vi "Run ESC Flight Profile.vi"(9 "Flight Profile File":path, 10 "Simulate/Run":T1=enum."Run VI", 11 "RPM PWM Calib File":path) -> (0 "error IO":errorcluster, 1 "Flight Profile Out":path)   [LabVIEW 2021]
uses:
  Anemometry/Anemometry Sub Vis/Controls/User_Specific_mode.ctl
  Anemometry/Anemometry Sub Vis/Controls/Inst_type.ctl
  Anemometry/Anemometry Sub Vis/Gen Trav/Multi_Run_Status.ctl
  Anemometry/Anemometry Sub Vis/Globals/Trav_pos_global.vi
  Anemometry/Anemometry Sub Vis/Globals/Meas_global.vi
panel:
  out "PWM":dbl format="%.2f"
  out "Time (s)":dbl[](array[numeric])
  out "Calib Constants":dbl[](array[numeric])
  out "XY Graph":cluster{dbl[], dbl[]}(graph)
  out "RPM":dbl[](array[numeric])
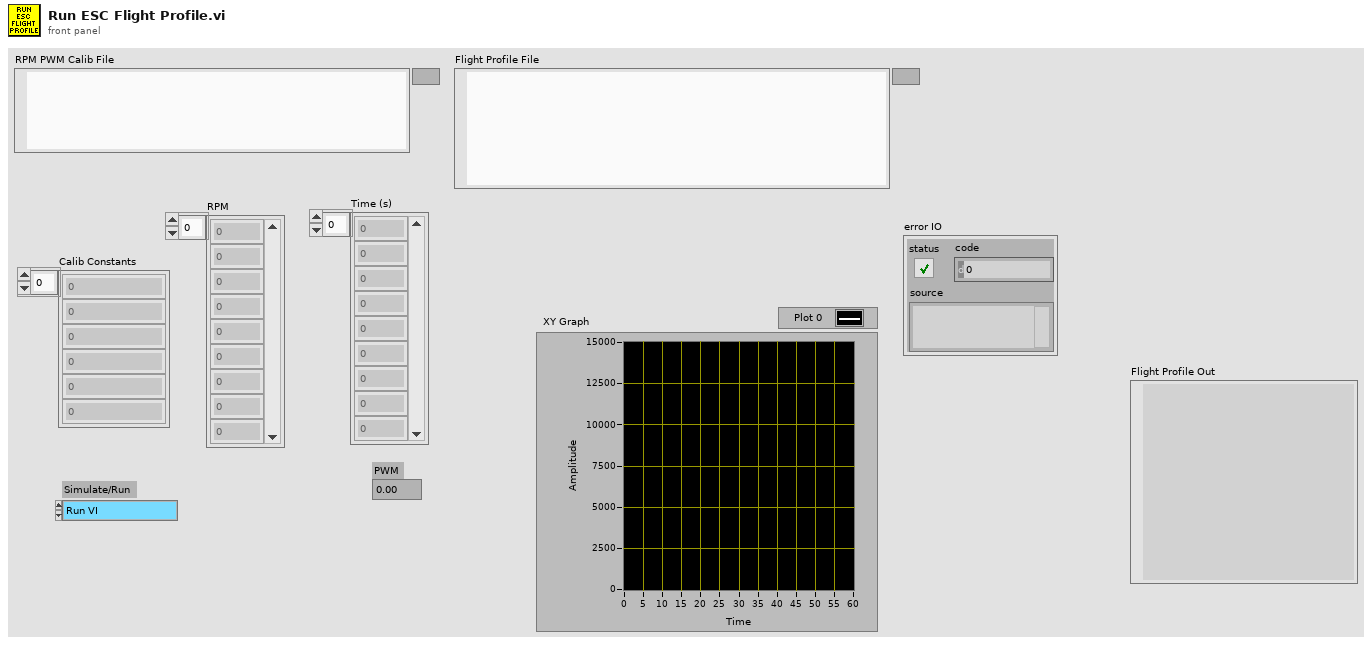
[diagram p1: front panel]
types:
  T1 = typedef "User_Specific_mode.ctl" = enum16{"Check VI only", "Run VI"}
  T2 = typedef "Inst_type.ctl" = enum16{"Raw voltage", "Raw with zero offsetting", "Propeller anemometer", "Pressure Transducer", "Pitot-static tube", "Hot wire", "Cross wire 1", "Cross wire 2", "Generic Linear", "Generic Polynomial", "Generic BackPoly", "Fast FID", "Thermocouple", "Cold wire", "Pulsed Wire", "LDA Vel", "LDA Tran time", "LDA Arr time", "Microphone"}
  T3 = typedef "Multi_Run_Status.ctl" = enum16{"Continue", "Continue with Error", "Jump to Next Point", "Jump to Next Row", "Jump To Fall Back", "Terminate Run"}
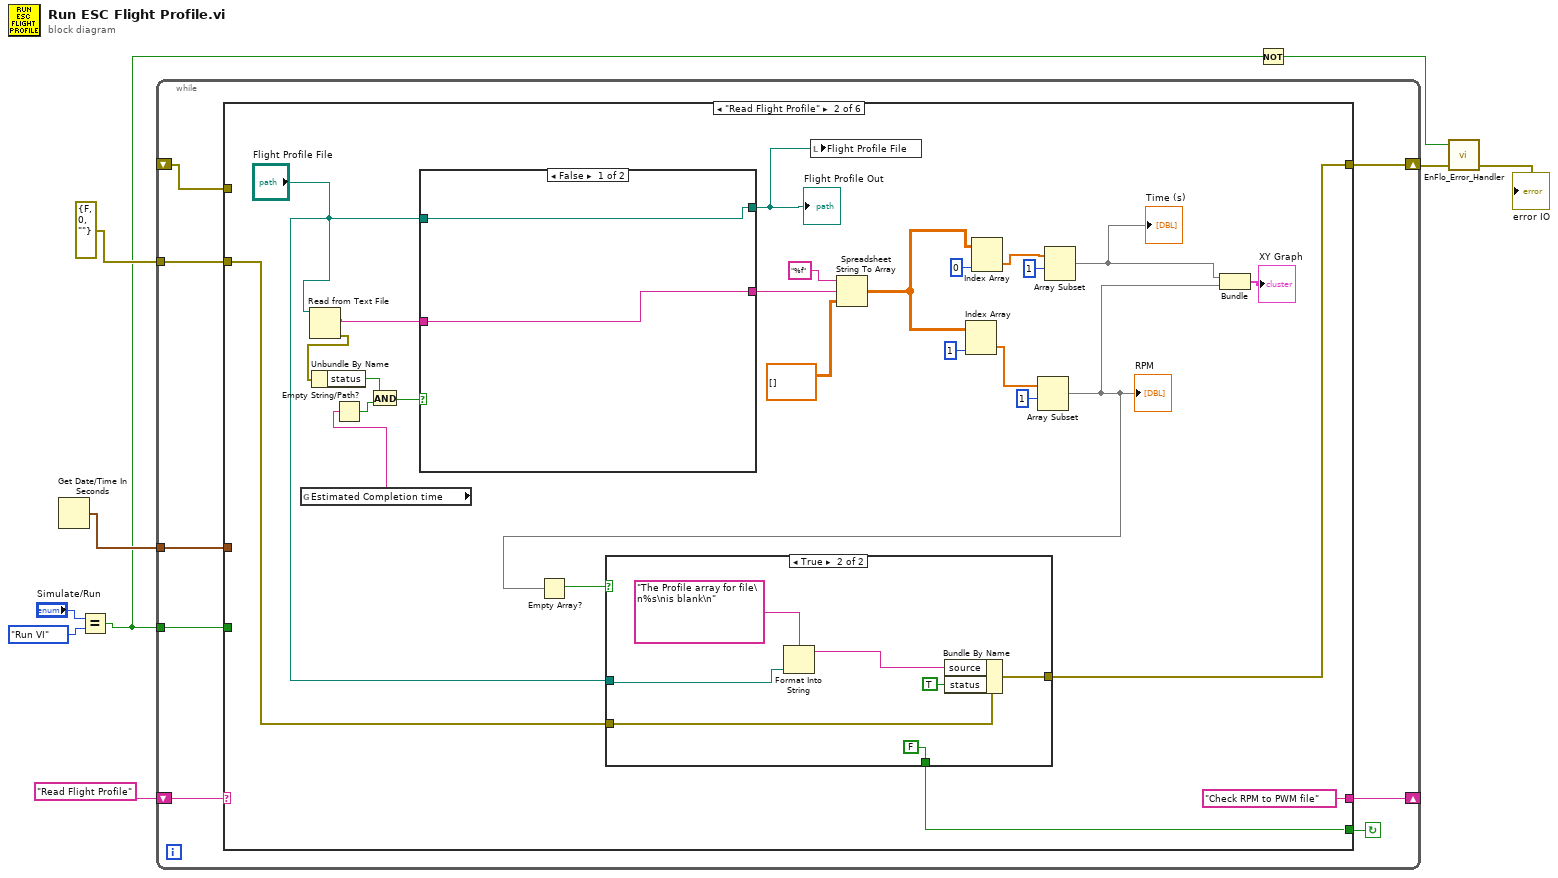
[diagram p0: block diagram]
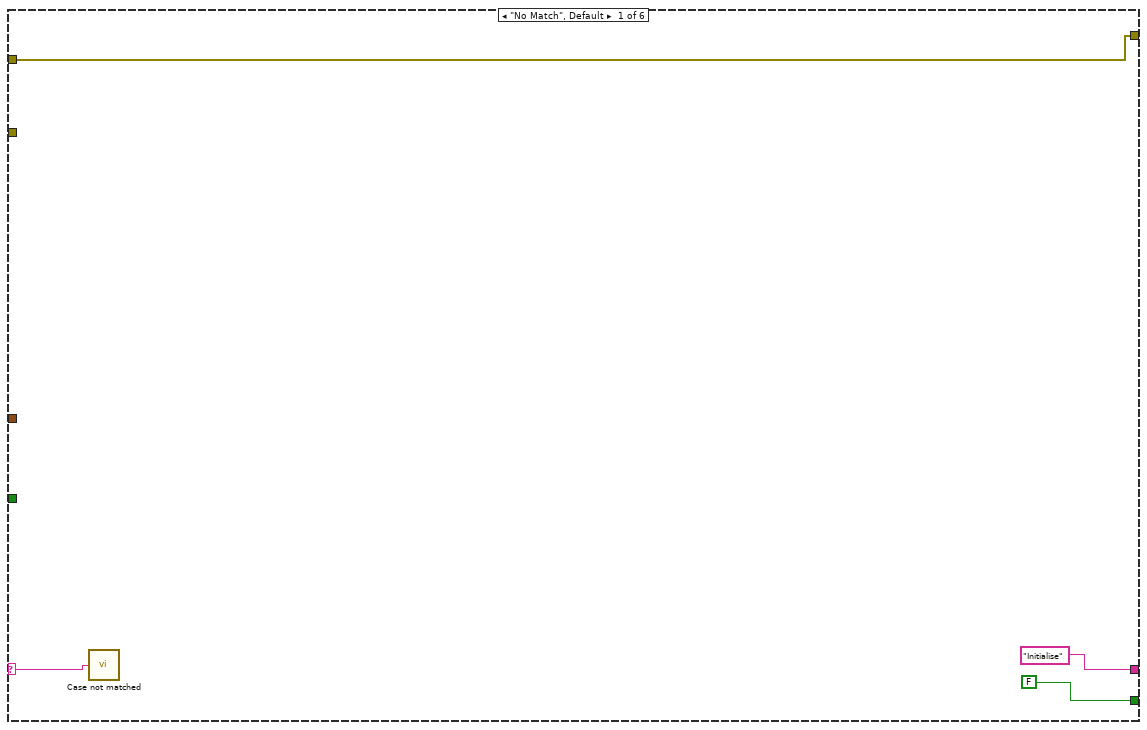
[diagram p2: hidden frame]
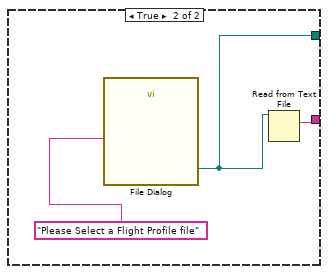
[diagram p3: hidden frame]
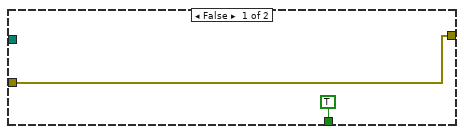
[diagram p4: hidden frame]
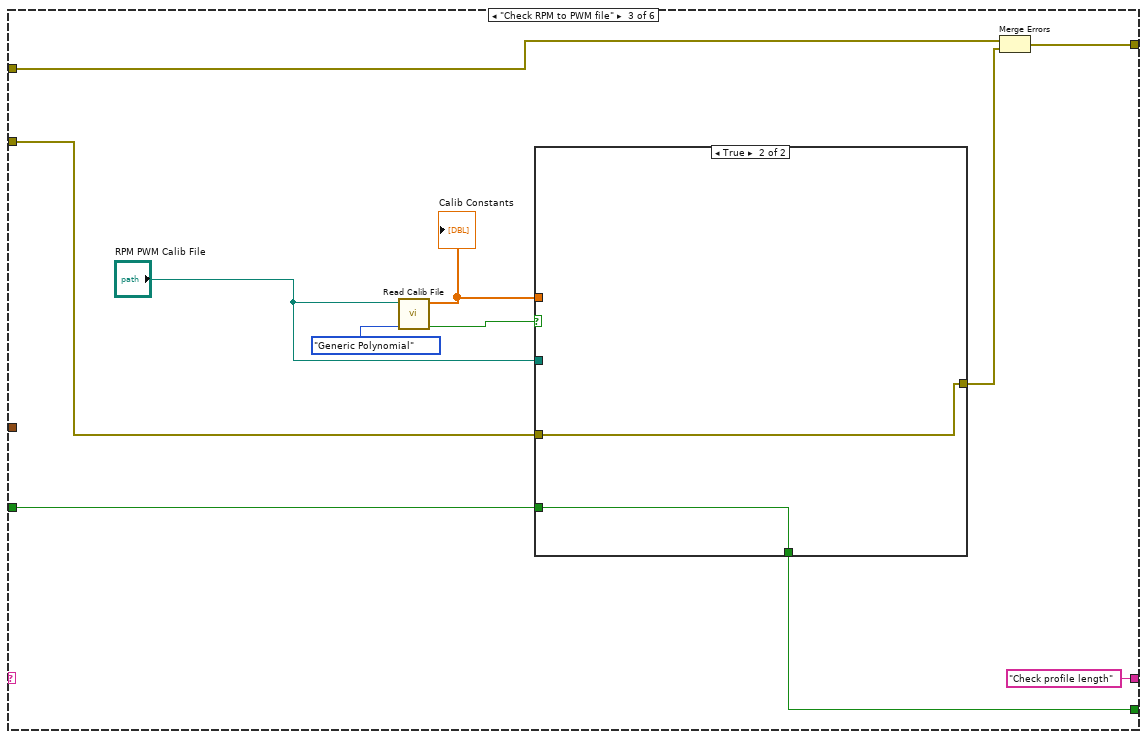
[diagram p5: hidden frame]
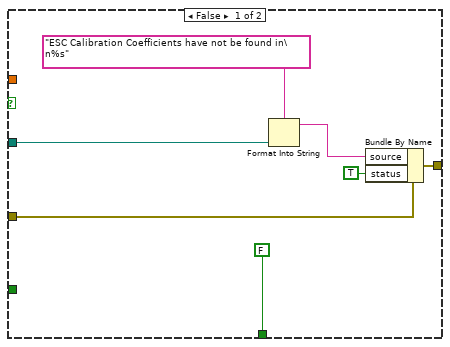
[diagram p6: hidden frame]
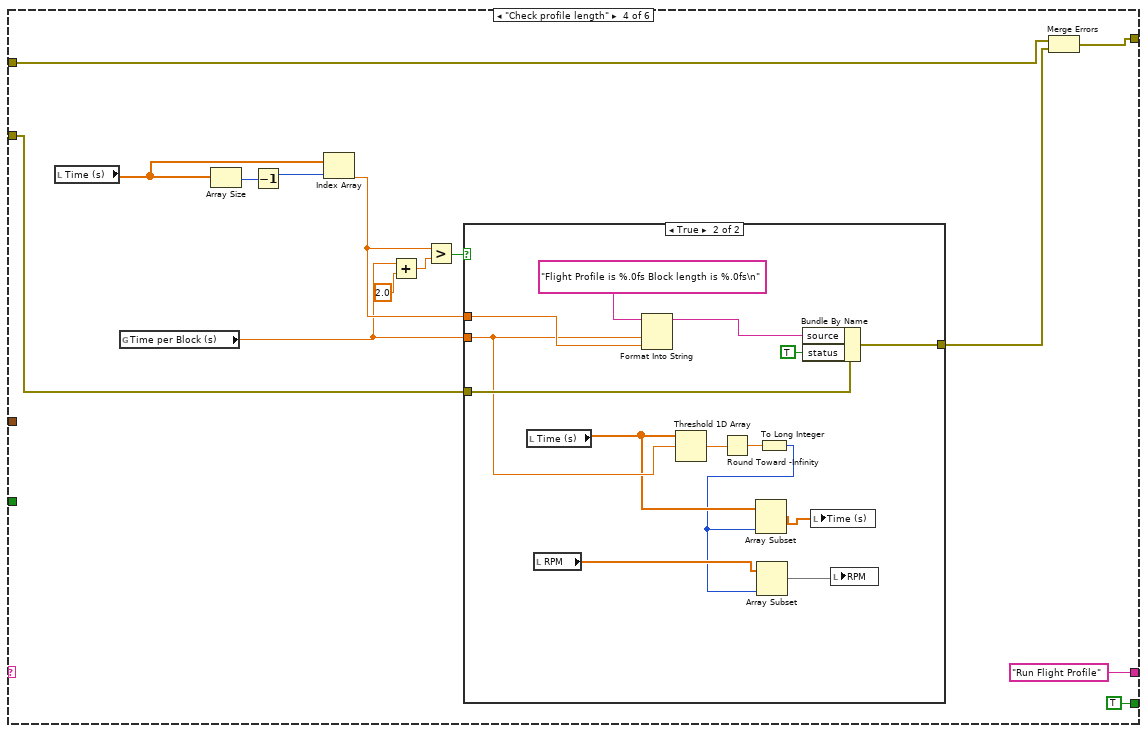
[diagram p7: hidden frame]
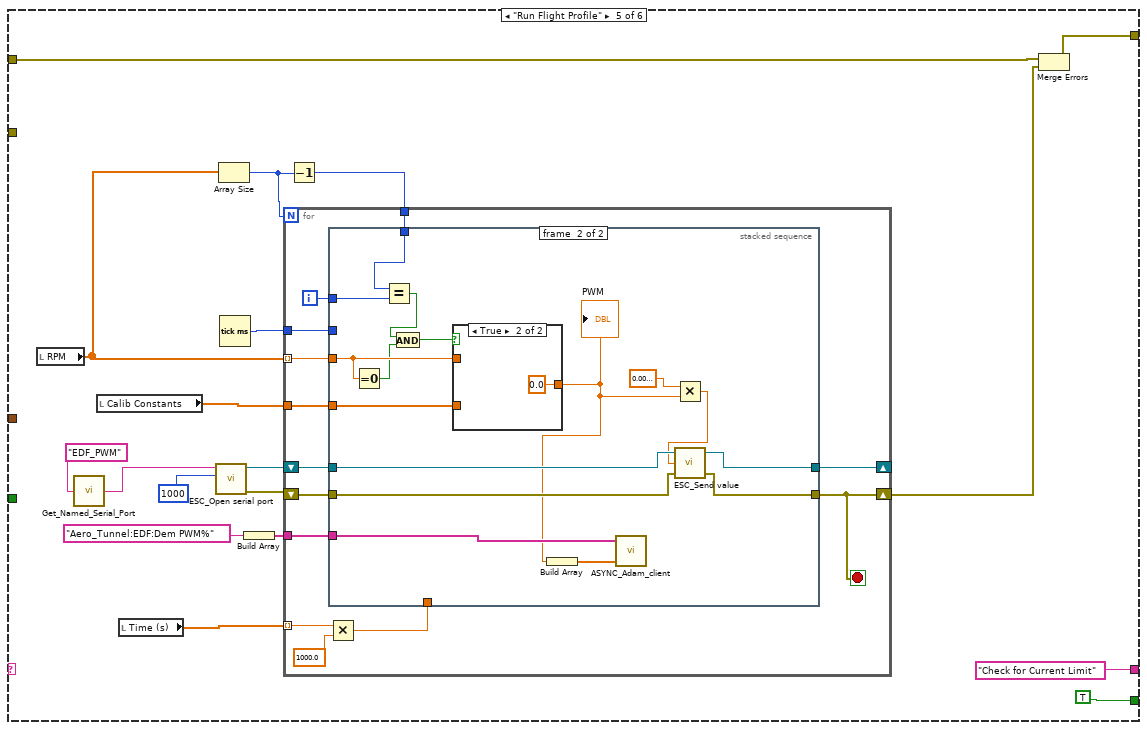
[diagram p9: hidden frame]
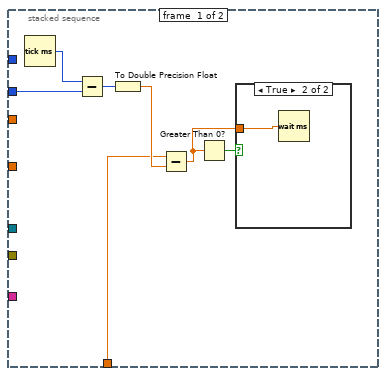
[diagram p10: hidden frame]
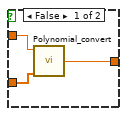
[diagram p12: hidden frame]
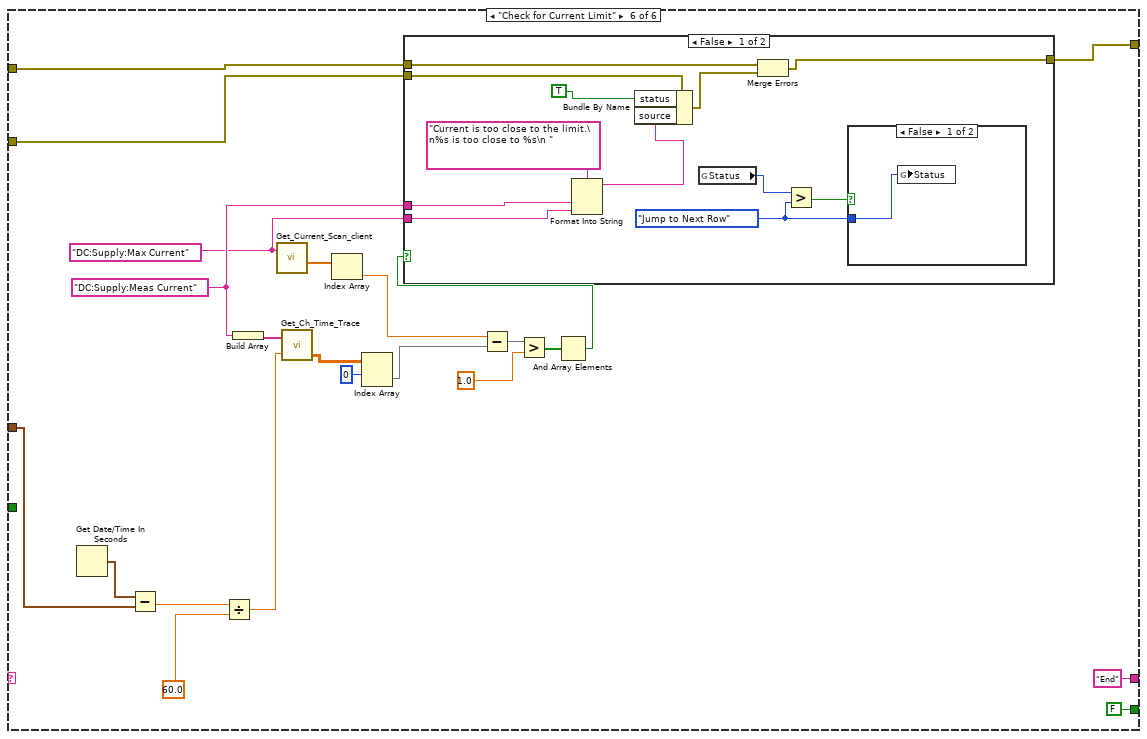
[diagram p13: hidden frame]
diagram:
  n1 = Get Date/Time In Seconds() -> (seconds since 1Jan1904=w7:timestamp)
  n2 = Equal?(x="Simulate/Run", y=User_Specific_mode."Run VI" ("Simulate/Run")) -> (x = y?=w2:bool)
  n3 = while {
    shift-left: "Read Flight Profile" -> [w14]
    shift-right: [w15] -> _
    tunnel: w7 -> [w13]
    tunnel: errorcluster {"status"=FALSE, "code"=0, "source"=""} ("error in (no error)") -> [w12]
    shift-right: [w11] -> w5
    shift-left: _ -> [w10]
    tunnel: w2 -> [w9]
    stop <- w16 continue-if-true
    n4 = case shown="\"Read Flight Profile\"" w14 {
      selector: w14 -> [w18 _ _ _ _ _]
      tunnel: [FALSE w34 w66 TRUE TRUE FALSE] -> w16
      tunnel: ["Initialise" "Check RPM to PWM file" "Check profile length" "Run Flight Profile" "Check for Current Limit" "End"] -> w15
      tunnel: w13 -> [_ _ _ _ _ w186]
      tunnel: w12 -> [_ w31 w64 w87 _ w171]
      tunnel: [w17 w30 w63 w84 w110 w169] -> w11
      tunnel: w10 -> [w17 _ w62 w85 w111 w170]
      tunnel: w9 -> [_ _ w61 _ _ _]
      frame "No Match", Default {
        n5 = call "Case not matched.vi"("Case Name not Matched"=w18) -> ()
      }
      frame "Read Flight Profile" {
        n6 = global read "Trav_pos_global.vi" "Estimated Completion time"() -> (w26:string)
        n7 = Read from Text File(file (use dialog)="Flight Profile File") -> (text=w23:string, error out=w29:errorcluster)  [unwired: 3 in, 2 out]
        n8 = Unbundle By Name(w29) -> ("status"=w28:bool)
        n9 = Empty String/Path?(string/path=w26) -> (empty?=w27:bool)
        n10 = And(x=w28, y=w27) -> (x .and. y?=w25:bool)
        n11 = case shown="False" w25 {
          tunnel: [w48 w50] -> w24
          tunnel: w23 -> [w48 _]
          tunnel: [w47 w49] -> w21
          tunnel: "Flight Profile File" -> [w47 _]
          frame False {
          }
          frame True {
            n12 = call "File Dialog"("prompt"="Please Select a Flight Profile file") -> ("selected path"=w49:path)  [unwired: 11 in, 3 out]
            n13 = Read from Text File(file (use dialog)=w49) -> (text=w50:string)  [unwired: 3 in, 3 out]
          }
        }
        "Flight Profile Out" <- w21
        n14 = local write "Flight Profile File"(w21) -> ()
        n15 = Spreadsheet String To Array(format string="%f", spreadsheet string=w24, array type (2D Dbl)=dbl[][] []) -> (array=w45:dbl[][])  [unwired: 1 in]
        n16 = Index Array(array=w45, index (col)=1 ("disabled index (col)")) -> (element=w44:dbl[])  [unwired: 1 in]
        n17 = Index Array(array=w45, index (col)=0 ("disabled index (col)")) -> (element=w46:dbl[])  [unwired: 1 in]
        n18 = Array Subset(array=w44, index=1) -> (w36:dbl[])  [unwired: 1 in]
        "RPM" <- w36
        n19 = Empty Array?(array=w36) -> (empty?=w35:bool)
        n20 = case shown="True" w35 {
          tunnel: [TRUE FALSE] -> w34
          tunnel: "Flight Profile File" -> [_ w59]
          tunnel: w31 -> [w52 w57]
          tunnel: [w52 w54] -> w30
          frame False {
          }
          frame True {
            n21 = Format Into String(format string="The Profile array for file\n%s\nis blank\n", w59) -> (resulting string=w55:string)  [unwired: 2 in, 1 out]
            n22 = Bundle By Name(cluster=w57, "source"=w55, "status"=TRUE) -> (w54:errorcluster)
          }
        }
        n23 = Array Subset(array=w46, index=1) -> (w32:dbl[])  [unwired: 1 in]
        "Time (s)" <- w32
        n24 = Bundle(w32, w36) -> (→"XY Graph":cluster{dbl[], dbl[]})  [unwired: 1 in]
      }
      frame "Check RPM to PWM file" {
        n25 = call "Read Calib File.vi"("Inst type"=Inst_type."Generic Polynomial", "Calib File"="RPM PWM Calib File") -> ("Coefficients Found?"=w68:bool, "Calib Constants"=w69:dbl[])  [unwired: 8 in]
        "Calib Constants" <- w69
        n26 = case shown="True" w68 {
          tunnel: w69 -> [_ _]
          tunnel: "RPM PWM Calib File" -> [w78 _]
          tunnel: [FALSE w79] -> w66
          tunnel: [w73 w80] -> w65
          tunnel: w64 -> [w72 w80]
          tunnel: w61 -> [_ w79]
          frame False {
            n27 = Format Into String(format string="ESC Calibration Coefficients have not be found in\n%s", w78) -> (resulting string=w74:string)  [unwired: 2 in, 1 out]
            n28 = Bundle By Name(cluster=w72, "source"=w74, "status"=TRUE) -> (w73:errorcluster)
          }
          frame True {
          }
        }
        n29 = Merge Errors(w62, w65) -> (w63:errorcluster)
      }
      frame "Check profile length" {
        n30 = local read "Time (s)"() -> (w90:dbl[])
        n31 = global read "Meas_global.vi" "Time per Block (s)"() -> (w83:dbl)
        n32 = Array Size(array=w90) -> (size(s)=w92:i32)
        n33 = Decrement(x=w92) -> (x-1=w91:i32)
        n34 = Index Array(array=w90, index=w91) -> (element=w88:dbl)
        n35 = Add(x=w83, y=2.0) -> (x+y=w82:dbl)
        n36 = Greater?(x=w88, y=w82) -> (0:w89:bool)
        n37 = case shown="True" w89 {
          tunnel: w87 -> [w95 w109]
          tunnel: [w95 w106] -> w86
          tunnel: w83 -> [_ w101]
          tunnel: w88 -> [_ w105]
          frame False {
          }
          frame True {
            n38 = local read "Time (s)"() -> (w100:dbl[])
            n39 = local read "RPM"() -> (w99:dbl[])
            n40 = Format Into String(format string="Flight Profile is %.0fs Block length is %.0fs\n", w101, w105) -> (resulting string=w107:string)  [unwired: 2 in, 1 out]
            n41 = Threshold 1D Array(2:w101, 3:w100) -> (0:w103:dbl)  [unwired: 1 in]
            n42 = Round Toward -Infinity(1:w103) -> (0:w102:dbl)
            n43 = To Long Integer(number=w102) -> (32bit integer=w98:i32)
            n44 = Array Subset(array=w100, length=w98) -> (w96:dbl[])  [unwired: 1 in]
            n45 = Array Subset(array=w99, length=w98) -> (w97:dbl[])  [unwired: 1 in]
            n46 = Bundle By Name(cluster=w109, "source"=w107, "status"=TRUE) -> (w106:errorcluster)
            n47 = local write "Time (s)"(w96) -> ()
            n48 = local write "RPM"(w97) -> ()
          }
        }
        n49 = Merge Errors(w85, w86) -> (w84:errorcluster)
      }
      frame "Run Flight Profile" {
        n50 = local read "RPM"() -> (w122:dbl[])
        n51 = call "Get_Named_Serial_Port.vi"("Serial Port Alias"="EDF_PWM") -> ("Serial Port Name"=w117:string)
        n52 = local read "Calib Constants"() -> (w123:dbl[])
        n53 = local read "Time (s)"() -> (w124:dbl[])
        n54 = call "ESC_Open serial port.vi"("timeout (ms)"=u32 1000, "VISA resource name"=w117) -> ("Error out"=w115:errorcluster, "VISA resource name out"=w116:refnum<visa-resource-name>)  [unwired: 8 in]
        n55 = Array Size(array=w122) -> (size(s)=w121:i32)
        n56 = Tick Count (ms)() -> (millisecond timer value=w125:u32)
        n57 = Build Array("Aero_Tunnel:EDF:Dem PWM%") -> (w113:string[])
        n58 = Decrement(x=w121) -> (x-1=w120:i32)
        n59 = for {
          N: w121 -> [_]
          tunnel: w125 -> [w140]
          tunnel: w124 -> [w139] mode=indexing
          tunnel: w123 -> [w136]
          tunnel: w122 -> [w135] mode=indexing
          tunnel: w120 -> [w134]
          shift-right: [w131] -> _
          shift-left: w116 -> [w132]
          shift-right: [w130] -> w112
          shift-left: w115 -> [w129]
          tunnel: w113 -> [w128]
          i -> [w133]
          stop <- w130 stop-if-true
          n60 = Multiply(x=w139, y=1000.0) -> (x*y=w137:dbl)
          n61 = stacked-sequence {
            tunnel: w140 -> [w146 _]
            tunnel: w137 -> [w141 _]
            tunnel: w136 -> [_ w164]
            tunnel: w135 -> [_ w163]
            tunnel: w134 -> [_ w161]
            tunnel: w133 -> [_ w160]
            tunnel: w132 -> [_ w156]
            tunnel: [_ w155] -> w130
            tunnel: [_ w154] -> w131
            tunnel: w129 -> [_ w153]
            tunnel: w128 -> [_ w152]
            frame #0 {
              n62 = Tick Count (ms)() -> (millisecond timer value=w147:u32)
              n63 = Subtract(x=w147, y=w146) -> (x-y=w145:u32)
              n64 = To Double Precision Float(number=w145) -> (double precision float=w144:dbl)
              n65 = Subtract(x=w141, y=w144) -> (x-y=w142:dbl)
              n66 = Greater Than 0?(x=w142) -> (x > 0?=w143:bool)
              n67 = case shown="True" w143 {
                tunnel: w142 -> [_ w148]
                frame False {
                }
                frame True {
                  n68 = Wait (ms)(milliseconds to wait=w148) -> ()  [unwired: 1 out]
                }
              }
            }
            frame #1 {
              n69 = Equal To 0?(x=w163) -> (x = 0?=w162:bool)
              n70 = Equal?(x=w161, y=w160) -> (x = y?=w159:bool)
              n71 = And(x=w159, y=w162) -> (x .and. y?=w158:bool)
              n72 = case shown="True" w158 {
                tunnel: w164 -> [w167 _]
                tunnel: w163 -> [w166 _]
                tunnel: [w165 0.0 ("Eng Values")] -> w149
                frame False {
                  n73 = call "Polynomial_convert.vi"("Calib constants"=w167, "Voltage"=w166) -> ("Eng Values"=w165:dbl)  [unwired: 4 out]
                }
                frame True {
                }
              }
              "PWM" <- w149
              n74 = Build Array(w149) -> (w150:dbl[])
              n75 = call "ASYNC_Adam_client.vi"("Values"=w150, "Channel Names"=w152) -> ()  [unwired: 1 in, 2 out]
              n76 = Multiply(x=sgl 0.01, y=w149) -> (x*y=w151:dbl)
              n77 = call "ESC_Send value.vi"("Error In"=w153, "Output (0...1)"=w151, "Port"=w156) -> ("Error Out"=w155:errorcluster, "Port out"=w154:refnum<visa-resource-name>)  [unwired: 1 out]
            }
          }
        }
        n78 = Merge Errors(w111, w112) -> (w110:errorcluster)
      }
      frame "Check for Current Limit" {
        w172 = "DC:Supply:Max Current" ("string")
        w173 = "DC:Supply:Meas Current"
        n79 = Get Date/Time In Seconds() -> (seconds since 1Jan1904=w187:timestamp)
        n80 = Subtract(x=w187, y=w186) -> (x-y=w185:dbl)
        n81 = Divide(x=w185, y=60.0) -> (x/y=w183:dbl)
        n82 = Build Array(w173) -> (w188:string[])
        n83 = call "Get_Current_Scan_client.vi"("singleChannel"=w172) -> ("Numerical Values"=w182:dbl[])  [unwired: 1 in, 3 out]
        n84 = call "Get_Ch_Time_Trace.vi"("Desired Ch Names"=w188, "History Length (mins)"=w183) -> ("Output array"=w179:dbl[][])  [unwired: 2 out]
        n85 = Index Array(array=w182) -> (element=w176:dbl)  [unwired: 1 in]
        n86 = Index Array(array=w179, index (row)=0) -> (element=w177:dbl[])  [unwired: 1 in]
        n87 = Subtract(x=w176, y=w177) -> (x-y=w180:dbl[])
        n88 = Greater?(x=w180, y=1.0) -> (0:w175:bool[])
        n89 = And Array Elements(Boolean array=w175) -> (logical AND=w174:bool)
        n90 = case shown="False" w174 {
          tunnel: w173 -> [w201 _]
          tunnel: w172 -> [w195 _]
          tunnel: w171 -> [w194 _]
          tunnel: w170 -> [w193 w204]
          tunnel: [w191 w204] -> w169
          frame False {
            w196 = Multi_Run_Status."Jump to Next Row" ("Status")
            n91 = Format Into String(format string="Current is too close to the limit.\n%s is too close to %s\n ", w201, w195) -> (resulting string=w199:string)  [unwired: 2 in, 1 out]
            n92 = Bundle By Name(cluster=w194, "status"=TRUE, "source"=w199) -> (w192:errorcluster)
            n93 = global read "Meas_global.vi" "Status"() -> (w198:T3)
            n94 = Merge Errors(w193, w192) -> (w191:errorcluster)
            n95 = Greater?(x=w198, y=w196) -> (0:w197:bool)
            n96 = case shown="False" w197 {
              tunnel: w196 -> [w203 _]
              frame False {
                n97 = global write "Meas_global.vi" "Status"(w203) -> ()
              }
              frame True {
              }
            }
          }
          frame True {
          }
        }
      }
    }
  }
  "error IO" <- w5
  n98 = Not(x=w2) -> (.not. x?=w1:bool)
  n99 = call "EnFlo_Error_Handler.vi"("error in (no error)"=w5, "Dialog Box (F)"=w1) -> ()  [unwired: 2 in, 2 out]
